vi "FdxCmdRxUDPReadCvi.vi"(8 "error in":errorcluster, 9 "MsgCount":u32, 10 "UdpHandle":u32, 11 "InstrumentHandle_port":u32) -> (0 "error out":errorcluster, 1 "ReadBuffer":u8[](array[numeric]), 2 "UdpHandle  Out":u32, 3 "InstrumentHandle_port":u32, 4 "MsgRead":u32)   [LabVIEW 2020, in "AIM664LV.lvlib"]
doc: "This function reads data from a UDP connection oriented port."
uses:
  AIM664LV.lvlib
  AFDX_LibraryAdmin/FdxGlobalDllPath.vi
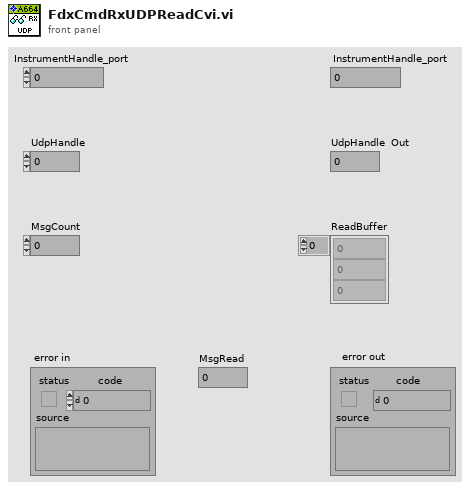
[diagram p1: front panel]
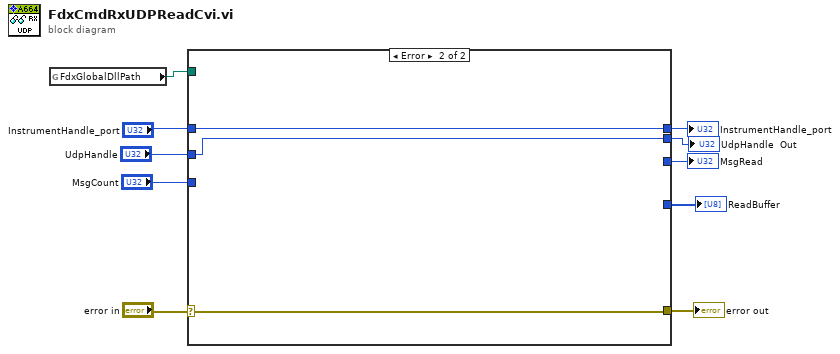
[diagram p0: block diagram]
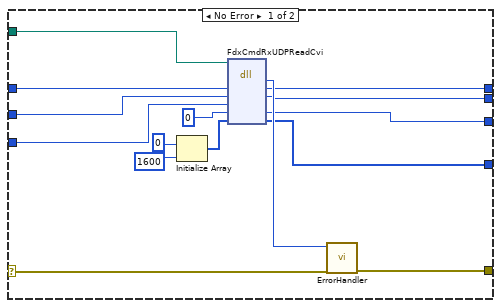
[diagram p2: hidden frame]
diagram:
  n1 = global read "FdxGlobalDllPath.vi" "FdxGlobalDllPath"() -> (w8:path)
  n2 = case shown="Error" "error in" {
    selector: "error in" -> [w24 w28]
    tunnel: [w25 w28] -> w10
    tunnel: w8 -> [w18 _]
    tunnel: "InstrumentHandle_port" -> [w17 w27]
    tunnel: [w16 w27] -> w6
    tunnel: "UdpHandle" -> [w15 w26]
    tunnel: "MsgCount" -> [w14 _]
    tunnel: [w13 _] -> w3
    tunnel: [w12 _] -> w2
    tunnel: [w11 w26] -> w1
    frame No Error {
      n3 = Initialize Array(u8 0 ("element"), 1600 ("dimension size")) -> (w20:u8[])
      n4 = dll-call lib="aim_fdx.19.dll" fn="FdxCmdRxUDPReadCvi"(path in=w18, "InstrumentHandle"=w17, "UdpHandle"=w15, "MsgCount"=w14, "MsgRead"=u32 0, "ReadBuffer"=w20) -> ("status"=w23:i32, "InstrumentHandle"=w16:u32, "UdpHandle"=w11:u32, "MsgRead"=w12:u32, "ReadBuffer"=w13:u8[])  [unwired: 3 in, 2 out]
      n5 = call "ErrorHandler.vi"("error in"=w24, "AIM Error"=w23) -> ("error out"=w25:errorcluster)  [unwired: 9 in]
    }
    frame Error {
    }
  }
  "error out" <- w10
  "InstrumentHandle_port" <- w6
  "ReadBuffer" <- w3
  "MsgRead" <- w2
  "UdpHandle  Out" <- w1
